vi "Login Failure.vi"(0 "Login View in":refnum<class "Login View.lvclass">, 5 "Login Message":string, 11 "error in (no error)":errorcluster) -> (4 "Login View out":refnum<class "Login View.lvclass">, 15 "error out":errorcluster)   [LabVIEW 2017, in "Login View.lvlib" / "Login View.lvclass"]
uses:
  Login View.lvclass
  Login View.lvclass/Login View.ctl
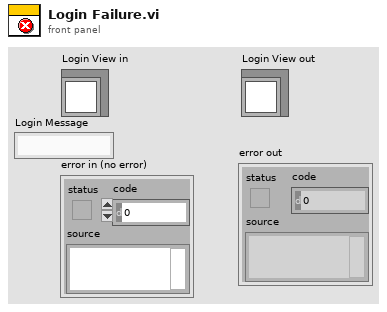
[diagram p1: front panel]
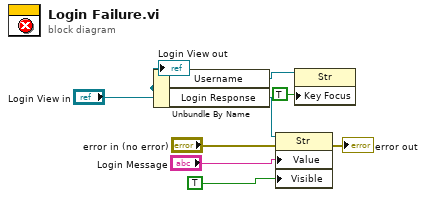
[diagram p0: block diagram]
diagram:
  n1 = Unbundle By Name("Login View in") -> ("Username"=w2:refnum<vi>, "Login Response"=w4:refnum<vi>)
  n2 = property on="Property Node" class="Str"(reference=w4, error in="error in (no error)", "Value"="Login Message", "Visible"=TRUE) -> (error out=→"error out":errorcluster)  [unwired: 1 out]
  n3 = property on="Property Node" class="Str"(reference=w2, "Key Focus"=TRUE) -> ()  [unwired: 1 in, 2 out]
  "Login View out" <- "Login View in"
